vi "convertAndAttachMetadata.vi"(8 "error in (no error)":errorcluster, 11 "experiment folder":path) -> (0 "error out":errorcluster, 3 "generated tdms file path":path)   [LabVIEW 2016]
uses:
  <userlib>/LevyLab/LV to ITX/Data/Typedefs/File Type--enum.ctl
  <userlib>/LevyLab/LV to ITX/Data/Data.lvclass
  <userlib>/LevyLab/LV to ITX/Macros/Conversion.lvclass
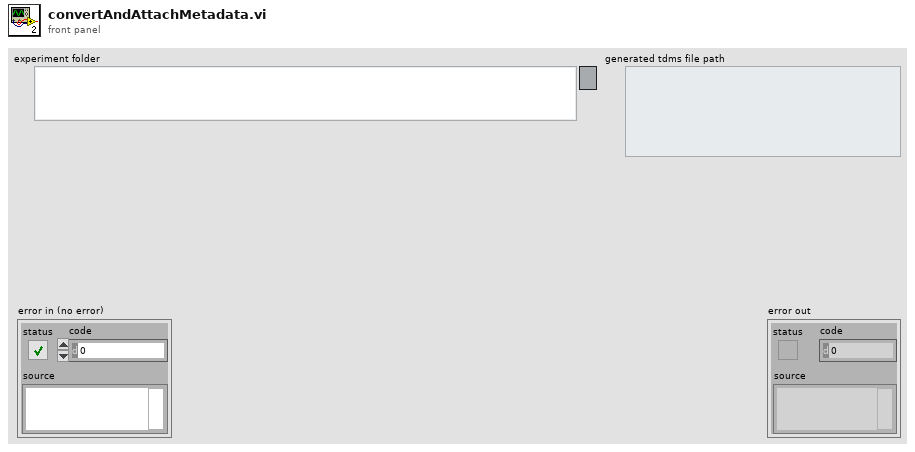
[diagram p1: front panel]
types:
  T1 = typedef "Data.lvclass/File Type--enum.ctl" = enum16{"DAT", "ITX", "TDMS", "VI"}
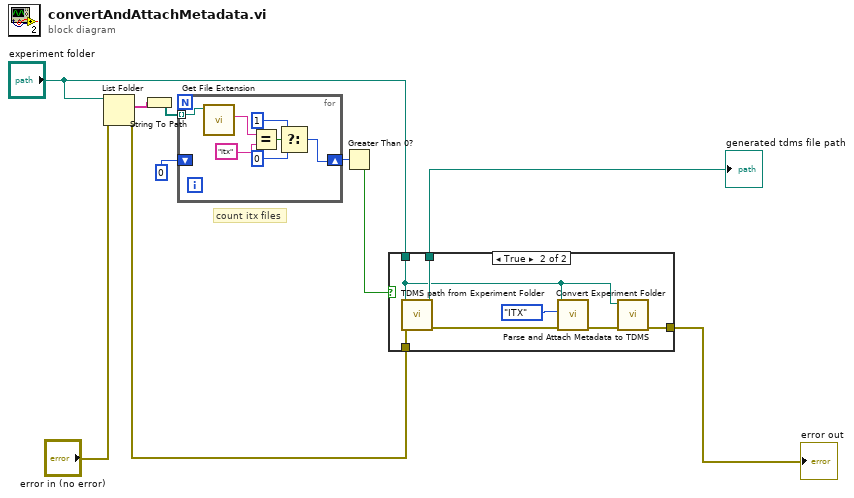
[diagram p0: block diagram]
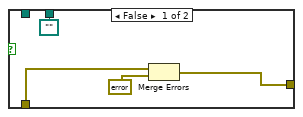
[diagram p2: hidden frame]
diagram:
  # "count itx files"
  n1 = List Folder(path="experiment folder", error in="error in (no error)") -> (filenames=w5:string[], error out=w6:errorcluster)  [unwired: 2 in, 2 out]
  n2 = String To Path(string=w5) -> (path=w4:path[])
  n3 = for {
    tunnel: w4 -> [w17] mode=indexing
    shift-right: [w11] -> w2
    shift-left: 0 ("f") -> [_]
    n4 = call <vilib>:"Get File Extension.vi"("file"=w17) -> ("lowercase file extension"=w16:string)  [unwired: 6 in, 4 out]
    n5 = Equal?(x=w16, y="itx") -> (x = y?=w14:bool)
    n6 = Select(t=1, s=w14, f=0) -> (s? t:f=w11:i32)
  }
  n7 = Greater Than 0?(x=w2) -> (x > 0?=w1:bool)
  n8 = case shown="True" w1 {
    tunnel: [path "" ("tdms file path") w27] -> w10
    tunnel: [w18 w24] -> w9
    tunnel: "experiment folder" -> [_ w23]
    tunnel: w6 -> [w20 w22]
    frame False {
      n9 = Merge Errors(w20, errorcluster {"status"=TRUE, "code"=44213, "source"="no itx files found"} ("error in")) -> (w18:errorcluster)
    }
    frame True {
      n10 = call "TDMS path from Experiment Folder.vi"("error in (no error)"=w22, "experiment folder"=w23) -> ("error out"=w26:errorcluster, "tdms file path"=w27:path)  [unwired: 7 in, 1 out]
      n11 = call <userlib>:"Convert Experiment Folder.vi"("error in (no error)"=w26, "Experiment Folder File Type"=File_Type--enum."ITX", "Experiment Folder Path"=w23) -> ("error out"=w25:errorcluster)  [unwired: 8 in]
      n12 = call "Parse and Attach Metadata to TDMS.vi"("error in (no error)"=w25, "experiment folder"=w23) -> ("error out"=w24:errorcluster)  [unwired: 8 in, 1 out]
    }
  }
  "generated tdms file path" <- w10
  "error out" <- w9
